vi "fpga_readout.vi"(0 "FPGA VI Reference In":refnum<k20>, 5 "samples":u64, 11 "error in":errorcluster) -> (4 "FPGA VI Reference Out":refnum<k20>, 6 "Voltage":dbl[][](array[numeric]), 8 "Counts":i16[][](array[numeric]), 10 "Interleaved Raw Data":u64[](array[numeric]), 15 "error out":errorcluster)   [LabVIEW 2015]
doc: "Reads out FPGA, deleaves and converts data to voltages. \nData is read out in 2000 elemnt increments as U64s. The data is deleaved into the individual channels and the counts are converted to voltages.\nThe ouput consists of a 32x[sample size] array of voltage, a 32x[sample size] array of raw counts and the raw 64 bit interleaved readout array."
uses:
  Controls/fpga_readout.ctl
  <instrlib>/_niInstr/Streaming/v1/Host/Public/Wait for Stream.vi
  <vilib>/Utility/error.llb/Error Cluster From Error Code.vi
  <vilib>/rvi/errors/niLvFpgaAdjustHostInterfaceError.vi
  <instrlib>/_niInstr/Streaming/v1/Host/Public/Start Finite Stream.vi
  <vilib>/rvi/interface/nirviReadWriteControl/nirviReadWriteControl.xnode
  <vilib>/rvi/interface/nirviMethod/nirviMethod.xnode
  <instrlib>/_niInstr/Streaming/v1/Host/niInstr Streaming v1 Host.lvlib
  <vilib>/rvi/interface/Simulation/niFpgaSimulationCallBeginRW.vi
  NiFpgaLv.dll
  <vilib>/FPGAPlugInAG/Dynamic/niLvFpga_ReadFifo_Dynamic.vi
  <vilib>/rvi/errors/niLvFpgaMergeErrorWithErrorCode.vi
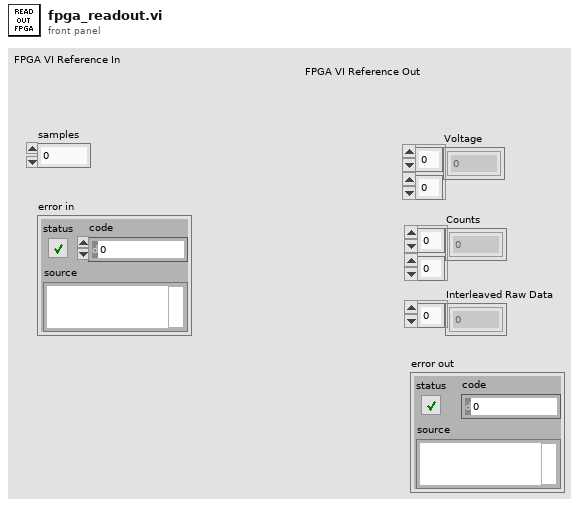
[diagram p1: front panel]
types:
  T1 = typedef "fpga_readout.ctl" = enum16{"determine DMA read cycles", "read", "deleave & convert to SI"}
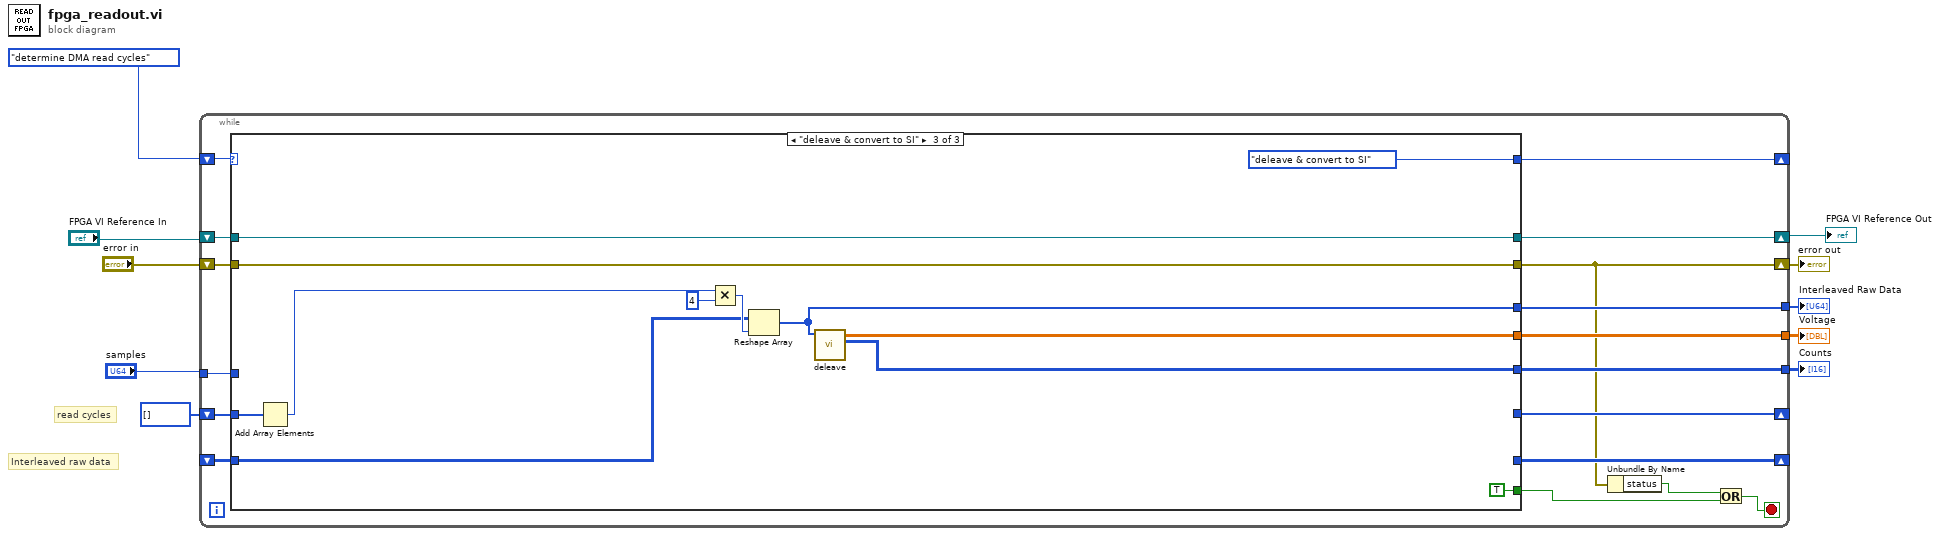
[diagram p0: block diagram]
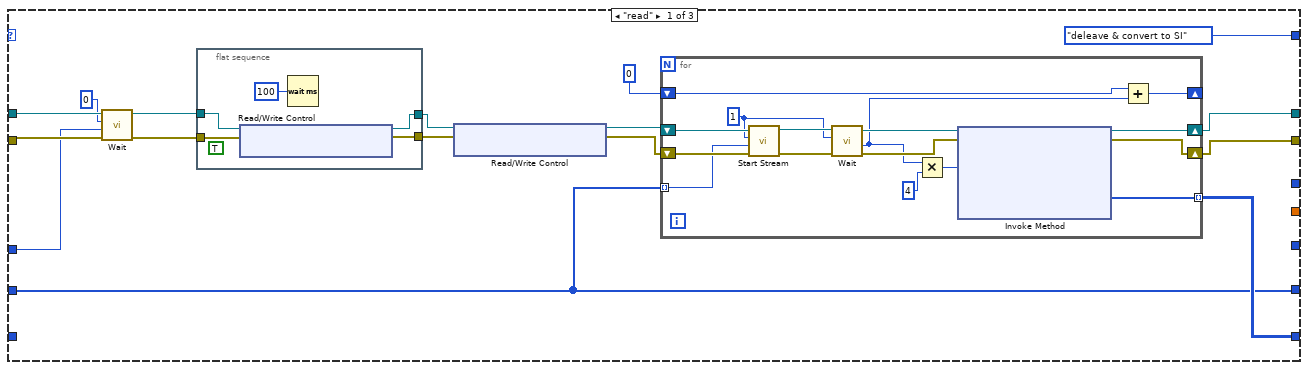
[diagram p2: hidden frame]
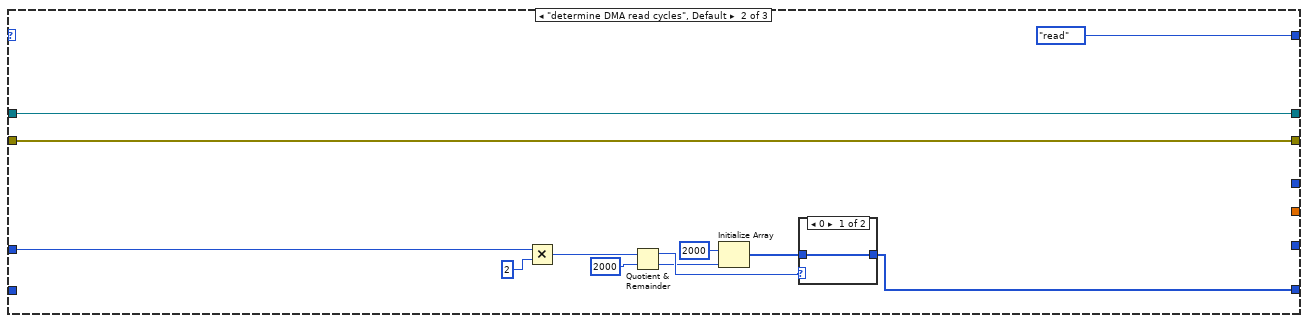
[diagram p3: hidden frame]
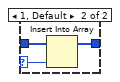
[diagram p4: hidden frame]
diagram:
  # "Interleaved raw data"
  # "read cycles"
  n1 = while {
    shift-right: [w21] -> w1
    shift-left: "FPGA VI Reference In" -> [w27]
    shift-right: [w12] -> w3
    shift-left: "error in" -> [w26]
    tunnel: "samples" -> [w25]
    shift-right: [w24] -> _
    shift-left: u64[] [] -> [w22]
    shift-right: [w20] -> _
    shift-left: _ -> [w19]
    tunnel: [w18] -> w6
    tunnel: [w17] -> w5
    tunnel: [w16] -> w4
    shift-right: [w15] -> _
    shift-left: fpga_readout."determine DMA read cycles" ("read out") -> [w23]
    stop <- w14 stop-if-true
    n2 = case shown="\"deleave & convert to SI\"" w23 {
      tunnel: w27 -> [w38 w66 w86]
      tunnel: w26 -> [w39 w67 w85]
      tunnel: w25 -> [w33 w69 _]
      tunnel: [w28 w68 _] -> w24
      tunnel: w22 -> [w28 _ w82]
      tunnel: [w32 w67 w85] -> w12
      tunnel: [w31 w66 w86] -> w21
      tunnel: [w30 _ _] -> w20
      tunnel: w19 -> [_ _ w90]
      tunnel: [_ _ w89] -> w18
      tunnel: [_ _ w88] -> w17
      tunnel: [_ _ w87] -> w16
      tunnel: [fpga_readout."deleave & convert to SI" ("read out") fpga_readout."read" ("read out") fpga_readout."deleave & convert to SI" ("read out")] -> w15
      tunnel: [_ _ TRUE] -> w13
      frame "read" {
        n3 = call-poly <instrlib>:"Wait.vi"("error in (no error)"=w39, "wait for samples transferred"=w33, "stream index"=0, "refnum in"=w38) -> ("error out"=w41:errorcluster, "refnum out"=w42:refnum<k20>)  [unwired: 4 in, 2 out]
        n4 = flat-sequence {
          tunnel: w41 -> [w64]
          tunnel: [w62] -> w40
          tunnel: w42 -> [w61]
          tunnel: [w60] -> w43
          frame #0 {
            (unwired) TRUE ("Reset DRAM write address")
            n5 = xnode "Read/Write Control"("FPGA VI Reference In"=w61, "error in"=w64) -> ("FPGA VI Reference Out"=w60:refnum<k20>, "error out"=w62:errorcluster)  [unwired: 1 in]
            n6 = Wait (ms)(milliseconds to wait=u32 100) -> ()  [unwired: 1 out]
          }
        }
        n7 = xnode "Read/Write Control"("FPGA VI Reference In"=w43, "error in"=w40) -> ("FPGA VI Reference Out"=w35:refnum<k20>, "error out"=w34:errorcluster)  [unwired: 1 in]
        n8 = for {
          shift-right: [w46] -> w31
          shift-left: w35 -> [w56]
          shift-right: [w45] -> w32
          shift-left: w34 -> [w55]
          shift-right: [w59] -> _
          shift-left: u64 0 -> [w52]
          tunnel: w28 -> [w53] mode=indexing
          tunnel: [w47] -> w30 mode=indexing
          w54 = 1 ("stream index")
          n9 = call-poly <instrlib>:"Start Stream.vi"("error in (no error)"=w55, "num samples"=w53, "stream index"=w54, "refnum in"=w56) -> ("error out"=w57:errorcluster, "refnum out"=w58:refnum<k20>)  [unwired: 6 in]
          n10 = call-poly <instrlib>:"Wait.vi"("error in (no error)"=w57, "stream index"=w54, "refnum in"=w58) -> ("error out"=w50:errorcluster, "samples transferred"=w49:u64, "refnum out"=w51:refnum<k20>)  [unwired: 5 in, 1 out]
          n11 = Multiply(x=w49, y=u64 4) -> (x*y=w44:u64)
          n12 = xnode "Invoke Method"("FPGA VI Reference In"=w51, "error in"=w50, "Number of Elements"=w44) -> ("FPGA VI Reference Out"=w46:refnum<k20>, "error out"=w45:errorcluster, "Data"=w47:u64[])  [unwired: 1 in, 1 out]
          n13 = Add(x=w52, y=w49) -> (x+y=w59:u64)
        }
      }
      frame "determine DMA read cycles", Default {
        n14 = Multiply(x=w69, y=u64 2) -> (x*y=w71:u64)
        n15 = Quotient & Remainder(x=w71, y=u64 2000) -> (x-y*floor(x/y)=w76:u64, floor(x/y)=w73:u64)
        n16 = Initialize Array(u64 2000 ("element"), w73) -> (w75:u64[])
        n17 = case shown="0" w76 {
          selector: w76 -> [_ w78]
          tunnel: w75 -> [w77 w80]
          tunnel: [w77 w79] -> w68
          frame 0 {
          }
          frame 1, Default {
            n18 = Insert Into Array(array=w80, new element=w78) -> (w79:u64[])  [unwired: 1 in]
          }
        }
      }
      frame "deleave & convert to SI" {
        n19 = Add Array Elements(numeric array=w82) -> (sum=w81:u64)
        n20 = Multiply(x=w81, y=u64 4) -> (x*y=w92:u64)
        n21 = Reshape Array(w90, w92) -> (w89:u64[])
        n22 = call "deleave.vi"("Data"=w89) -> ("Counts"=w87:i16[][], "Voltage"=w88:dbl[][])  [unwired: 9 in]
      }
    }
    n23 = Unbundle By Name(w12) -> ("status"=w11:bool)
    n24 = Or(x=w11, y=w13) -> (x .or. y?=w14:bool)
  }
  "Interleaved Raw Data" <- w6
  "Voltage" <- w5
  "Counts" <- w4
  "error out" <- w3
  "FPGA VI Reference Out" <- w1
